vi "Teleop.vi"   [LabVIEW 2013]
doc: "This VI is called for each TeleOp packet received from the DS where the robot is not disabled. It is often used to read from the joysticks and update I/O or to update setpoints for timed control loops. It should complete and return within 20 milliseconds or it may miss DS packets."
uses:
  <vilib>/Rock Robotics/WPI/RobotDrive/WPI_RobotDriveGetSetRefNum.vi
  <vilib>/Rock Robotics/WPI/Joystick/WPI_JoystickGetSetRefNum.vi
types:
  T1 = typedef "WPI_JoystickDevRef.ctl" = cluster{"Device":T2}
  T2 = typedef "WPI_JoystickDeviceEnum.ctl" = enum16{"USB 1", "USB 2", "USB 3", "USB 4", "Kinect 1", "Kinect 2"}
  T3 = typedef "WPI_JoystickButtonState.ctl" = cluster{"Button 1":bool, "Button 2":bool, "Button 3":bool, "Button 4":bool, "Button 5":bool, "Button 6":bool, "Button 7":bool, "Button 8":bool, "Button 9":bool, "Button 10":bool, "Button 11":bool, "Button 12":bool}
  T4 = cluster{"axis 1 (x)":dbl, "axis 2 (y)":dbl, "axis 3 (throttle)":dbl, "axis 4":dbl, "axis 5":dbl, "axis 6":dbl}
  T5 = typedef "WPI_RobotDriveDevRef.ctl" = cluster{"DevStatus":errorcluster, "Motors[]":T6[], "Square Inputs":bool, "Max Output":dbl, "Isochronous":bool}
  T6 = typedef "WPI_MotorControlDeviceRef.ctl" = cluster{"DeviceStatus":errorcluster, "Type":enum16{"PWM", "CAN"}, "PWM":cluster{"Digital Module":T7, "PWM Channel":T8, "DeadBand":T9}, "CAN":cluster{"Device Number":u8, "Control Mode":T10, "Semaphore":T11, "Max Vout":dbl}, "Invert":bool, "TransformRef":T12, "InvTransformRef":T12}
  T7 = typedef "FPGA_TypedefDigitalModule.ctl" = enum16{"Digital Module 1", "Digital Module 2"}
  T8 = typedef "FPGA_DIOPWMChannel.ctl" = enum8{"PWM 1", "PWM 2", "PWM 3", "PWM 4", "PWM 5", "PWM 6", "PWM 7", "PWM 8", "PWM 9", "PWM 10", "Invalid"}
  T9 = typedef "WPI_PWMDeadband.ctl" = cluster{"Name":string, "maxPositivePwm":i32, "minPositivePwm":i32, "centerPwm":i32, "maxNegativePwm":i32, "minNegativePwm":i32, "angularRange":u16}
  T10 = typedef "WPI_CANJaguar_ControlMode.ctl" = enum8{"Percent VBus", "Current", "Speed", "Position", "Voltage"}
  T11 = typedef "Semaphore RefNum" = refnum<k1>
  T12 = typedef "WPI_PWMTransform_ConPane.ctl" = refnum<vi>
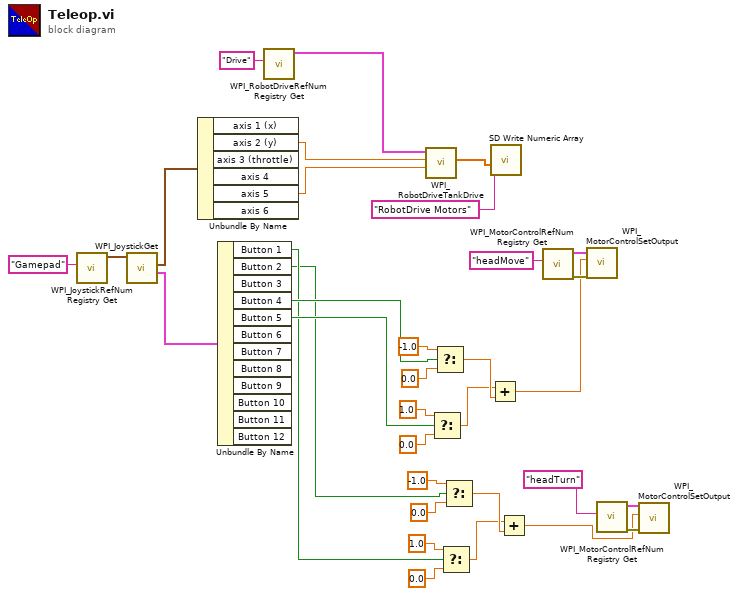
[diagram p0: block diagram]
diagram:
  n1 = call <vilib>:"WPI_JoystickRefNum Registry Get.vi"("refnum name"="Gamepad") -> ("JoystickDevRef"=w33:T1)  [unwired: 9 in, 1 out]
  n2 = call <vilib>:"WPI_JoystickGet.vi"("JoystickDevRef"=w33) -> ("Buttons"=w32:T3, "Axes"=w31:T4)  [unwired: 4 in, 1 out]
  n3 = Unbundle By Name(w31) -> ("axis 2 (y)"=w28:dbl, "axis 5"=w27:dbl)  [unwired: 4 out]
  n4 = Unbundle By Name(w32) -> ("Button 1"=w2:bool, "Button 2"=w1:bool, "Button 4"=w14:bool, "Button 5"=w13:bool)  [unwired: 8 out]
  n5 = call <vilib>:"WPI_RobotDriveRefNum Registry Get.vi"("refnum name"="Drive") -> ("RobotDriveDevRef"=w30:T5)  [unwired: 9 in, 1 out]
  n6 = call <vilib>:"WPI_RobotDriveTankDrive.vi"("Right axis value"=w27, "Left axis value"=w28, "RobotDriveDevRef"=w30) -> ("Motor Values"=w26:dbl[])  [unwired: 6 in, 2 out]
  n7 = Select(t=1.0, s=w13, f=0.0) -> (s? t:f=w11:dbl)
  n8 = Select(t=-1.0, s=w14, f=0.0) -> (s? t:f=w12:dbl)
  n9 = Select(t=1.0, s=w2, f=0.0) -> (s? t:f=w4:dbl)
  n10 = Select(t=-1.0, s=w1, f=0.0) -> (s? t:f=w5:dbl)
  n11 = Add(x=w11, y=w12) -> (x+y=w10:dbl)
  n12 = call <vilib>:"SD Write Numeric Array.vi"("Numeric Array"=w26, "Name"="RobotDrive Motors") -> ()  [unwired: 8 in, 2 out]
  n13 = Add(x=w4, y=w5) -> (x+y=w3:dbl)
  n14 = call <vilib>:"WPI_MotorControlRefNum Registry Get.vi"("refnum name"="headMove") -> ("error out"=w22:errorcluster, "MotorControlDevRef"=w21:T6)  [unwired: 9 in]
  n15 = call <vilib>:"WPI_MotorControlSetOutput.vi"("error in (no error)"=w22, "Output"=w10, "MotorControlDevRef"=w21) -> ()  [unwired: 6 in, 3 out]
  n16 = call <vilib>:"WPI_MotorControlRefNum Registry Get.vi"("refnum name"="headTurn") -> ("error out"=w20:errorcluster, "MotorControlDevRef"=w19:T6)  [unwired: 9 in]
  n17 = call <vilib>:"WPI_MotorControlSetOutput.vi"("error in (no error)"=w20, "Output"=w3, "MotorControlDevRef"=w19) -> ()  [unwired: 6 in, 3 out]
